vi "4p1_HW_Task2_fishele.vi"() -> ()   [LabVIEW 2021]
panel:
  out "Final Temperature":dbl=126.02264634930293
  in  "Unit Selector:":u16(ring) items=["Celsius", "Kelvin"]
  out "Ref temp in K":dbl=346.15
  in  "R0 Resistance at T0 (Ohms)":dbl=2081.0
  in  "T0 Ref. Temp (Celsius)":dbl=73.0
  in  "B thermal property (K)":dbl=2934.0
  in  "Resistance at current temp (Ohms)":dbl=675.0
  # "Inputs"
  # "Outputs"
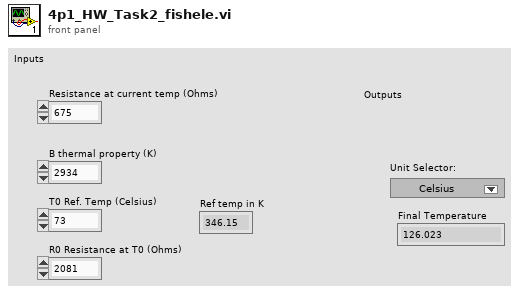
[diagram p1: front panel]
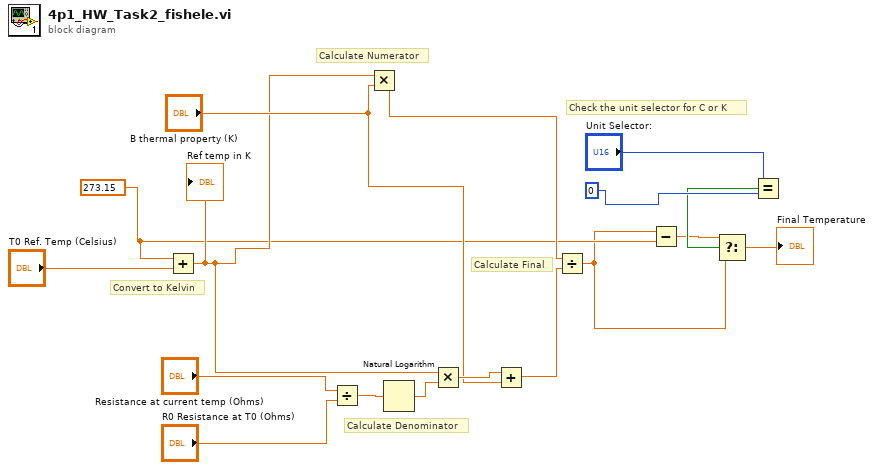
[diagram p0: block diagram]
diagram:
  w7 = 273.15 ("x")
  # "Calculate Final"
  # "Calculate Denominator"
  # "Calculate Numerator"
  # "Convert to Kelvin"
  # "Check the unit selector for C or K"
  n1 = Add(x=w7, y="T0 Ref. Temp (Celsius)") -> (x+y=w8:dbl)
  "Ref temp in K" <- w8
  n2 = Divide(x="Resistance at current temp (Ohms)", y="R0 Resistance at T0 (Ohms)") -> (x/y=w15:dbl)
  n3 = Multiply(x=w8, y="B thermal property (K)") -> (x*y=w11:dbl)
  n4 = Natural Logarithm(1:w15) -> (0:w14:dbl)
  n5 = Multiply(x=w8, y=w14) -> (x*y=w13:dbl)
  n6 = Add(x=w13, y="B thermal property (K)") -> (x+y=w10:dbl)
  n7 = Divide(x=w11, y=w10) -> (x/y=w1:dbl)
  n8 = Subtract(x=w1, y=w7) -> (x-y=w3:dbl)
  n9 = Equal?(x="Unit Selector:", y=u16 0) -> (x = y?=w4:bool)
  n10 = Select(t=w3, s=w4, f=w1) -> (s? t:f=→"Final Temperature":dbl)
